vi "RX-SIM-BPCS-UDP.vi"() -> ()   [LabVIEW 2017]
uses:
  <vilib>/Platform/TimedLoop/XDataNode/timing_clust.ctl
  <vilib>/Platform/TimedLoop/XDataNode/nitl_modes.ctl
  <vilib>/Platform/TimedLoop/XDataNode/wakeup.ctl
  <vilib>/Platform/TimedLoop/XDataNode/XDataNode.xnode
  <vilib>/Platform/TimedLoop/XDataNode/XDNodeRunTimeDep.lvlib
panel:
  in  "Stop":bool
  out "SIM-BPCS-RX-ARRAY":dbl[](array[numeric])
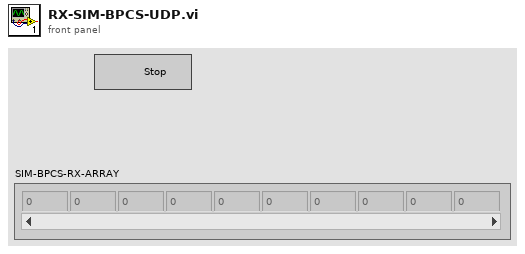
[diagram p1: front panel]
types:
  T1 = typedef "XDNodeRunTimeDep.lvlib/timing_clust.ctl" = cluster{"Expected End [f-1]":u64, "Actual End [f-1]":u64, "Finished Late? [f-1]":bool, "Expected End [i-1]":u64, "Actual End [i-1]":u64, "Finished Late? [i-1]":bool, "Expected Start [i]":u64, "Actual Start [i]":u64, "Expected Start [f]":u64, "Actual Start [f]":u64, "Source Name":string, "Structure Name":string, "Period":i64, "Deadline":i64, "Offset":i64, "Start":i64, "Priority":i32, "Timeout":i32, "Mode":T2, "Wakeup Reason":T3, "Error":errorcluster, "Source Type":string, "Secondary Source Type":string, "Global End Time":u64, "Global Start Time":u64, "Frame Duration":u64, "Iteration Duration":u64, "Assigned CPU":i32, "I/O Scan Engine Mode":u32}
  T2 = typedef "XDNodeRunTimeDep.lvlib/nitl_modes.ctl" = enum32{"No Change", "Process missed periods, maintain original phase", "Discard missed periods, maintain original phase", "Process missed periods, ignore original phase", "Discard missed periods, ignore original phase"}
  T3 = typedef "XDNodeRunTimeDep.lvlib/wakeup.ctl" = enum32{"Normal", "Aborted", "Asynchronous wakeup", "Timing source error", "Timed loop error", "Timeout"}
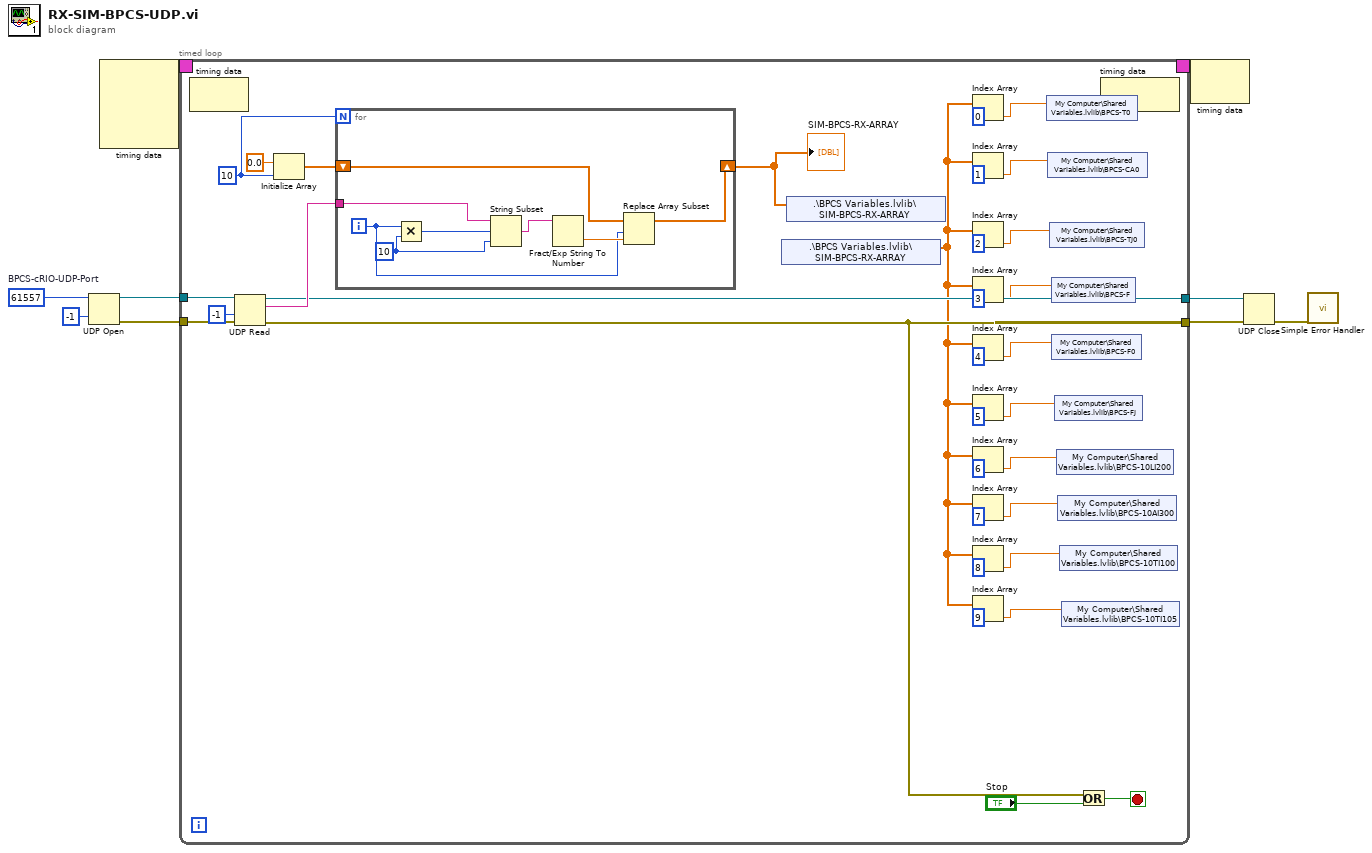
[diagram p0: block diagram]
diagram:
  w7 = u16 61557  # BPCS-cRIO-UDP-Port
  n1 = UDP Open(9:-1 ("timeout ms (25000)"), 11:w7) -> (port=w6:refnum<k16>, 0:w5:errorcluster)  [unwired: 3 in, 1 out]
  n2 = node-c288() -> (w9:T1)  [unwired: 4 in]
  n3 = timed-loop {
    timing: w9 -> [_]
    timing-out: [_] -> w8
    tunnel: w6 -> [w40]
    tunnel: w5 -> [w39]
    tunnel: [w37] -> w3
    tunnel: [w36] -> w2
    stop <- w41 stop-if-true
    w33 = 10 ("dimension size")
    n4 = node-c288() -> ()  [unwired: 1 in, 1 out]
    n5 = UDP Read(connection ID=w40, timeout ms (25000)=-1, 8:w39) -> (data out=w38:string, error out=w36:errorcluster, 3:w37:refnum<k16>)  [unwired: 3 out]
    n6 = Initialize Array(0.0 ("element"), w33) -> (w34:dbl[])
    n7 = for {
      N: w33 -> [_]
      tunnel: w38 -> [w49]
      shift-right: [w45] -> w32
      shift-left: w34 -> [w44]
      i -> [w46]
      w43 = 10 ("y")
      n8 = Multiply(x=w46, y=w43) -> (x*y=w48:i32)
      n9 = String Subset(string=w49, offset (0)=w48, length (rest)=w43) -> (substring=w50:string)
      n10 = Fract/Exp String To Number(string=w50) -> (number=w47:dbl)  [unwired: 3 in, 1 out]
      n11 = Replace Array Subset(array=w44, new element=w47, index=w46) -> (w45:dbl[])
    }
    "SIM-BPCS-RX-ARRAY" <- w32
    n12 = shared-variable ".\\BPCS Variables.lvlib\\SIM-BPCS-RX-ARRAY"() -> (w21:dbl[])  [unwired: 1 in, 1 out]
    n13 = shared-variable ".\\BPCS Variables.lvlib\\SIM-BPCS-RX-ARRAY"(w32) -> ()  [unwired: 1 in, 1 out]
    n14 = Index Array(array=w21, index=0) -> (element=w20:dbl)
    n15 = Index Array(array=w21, index=1) -> (element=w19:dbl)
    n16 = Index Array(array=w21, index=2) -> (element=w18:dbl)
    n17 = Index Array(array=w21, index=3) -> (element=w17:dbl)
    n18 = Index Array(array=w21, index=4) -> (element=w16:dbl)
    n19 = Index Array(array=w21, index=5) -> (element=w15:dbl)
    n20 = Index Array(array=w21, index=6) -> (element=w14:dbl)
    n21 = Index Array(array=w21, index=7) -> (element=w13:dbl)
    n22 = Index Array(array=w21, index=8) -> (element=w12:dbl)
    n23 = Index Array(array=w21, index=9) -> (element=w11:dbl)
    n24 = shared-variable "My Computer\\Shared Variables.lvlib\\BPCS-T0"(w20) -> ()  [unwired: 1 in, 1 out]
    n25 = shared-variable "My Computer\\Shared Variables.lvlib\\BPCS-CA0"(w19) -> ()  [unwired: 1 in, 1 out]
    n26 = shared-variable "My Computer\\Shared Variables.lvlib\\BPCS-TJ0"(w18) -> ()  [unwired: 1 in, 1 out]
    n27 = shared-variable "My Computer\\Shared Variables.lvlib\\BPCS-F"(w17) -> ()  [unwired: 1 in, 1 out]
    n28 = shared-variable "My Computer\\Shared Variables.lvlib\\BPCS-F0"(w16) -> ()  [unwired: 1 in, 1 out]
    n29 = shared-variable "My Computer\\Shared Variables.lvlib\\BPCS-FJ"(w15) -> ()  [unwired: 1 in, 1 out]
    n30 = shared-variable "My Computer\\Shared Variables.lvlib\\BPCS-10LI200"(w14) -> ()  [unwired: 1 in, 1 out]
    n31 = shared-variable "My Computer\\Shared Variables.lvlib\\BPCS-10AI300"(w13) -> ()  [unwired: 1 in, 1 out]
    n32 = shared-variable "My Computer\\Shared Variables.lvlib\\BPCS-10TI100"(w12) -> ()  [unwired: 1 in, 1 out]
    n33 = shared-variable "My Computer\\Shared Variables.lvlib\\BPCS-10TI105"(w11) -> ()  [unwired: 1 in, 1 out]
    n34 = Or(x=w36, y="Stop") -> (x .or. y?=w41:bool)
    n35 = node-c288() -> ()  [unwired: 1 in, 1 out]
  }
  n36 = node-c288(w8) -> ()  [unwired: 1 out]
  n37 = UDP Close(connection ID=w3, 8:w2) -> (error out=w4:errorcluster)  [unwired: 1 out]
  n38 = call <vilib>:"Simple Error Handler.vi"("error in (no error)"=w4) -> ()  [unwired: 4 in, 5 out]
